vi "FlushTcpPortBase.vi"(6 "max flush time (ms)":i32=5000, 8 "error in (no error)":errorcluster, 11 "tcp in":refnum<k5>) -> (0 "error out":errorcluster, 1 "timed out":bool, 2 "data flushed":bool, 3 "tcp out":refnum<k5>)   [LabVIEW 2017]
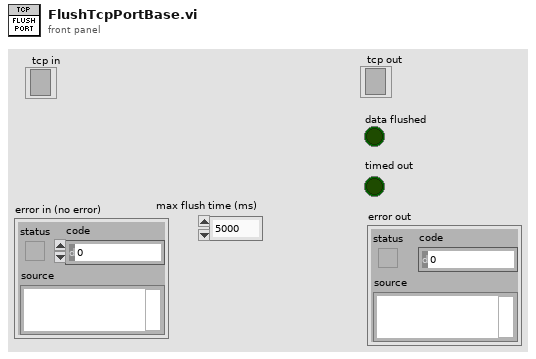
[diagram p1: front panel]
types:
  T1 = enum16{"Standard", "Buffered", "CRLF", "Immediate"}
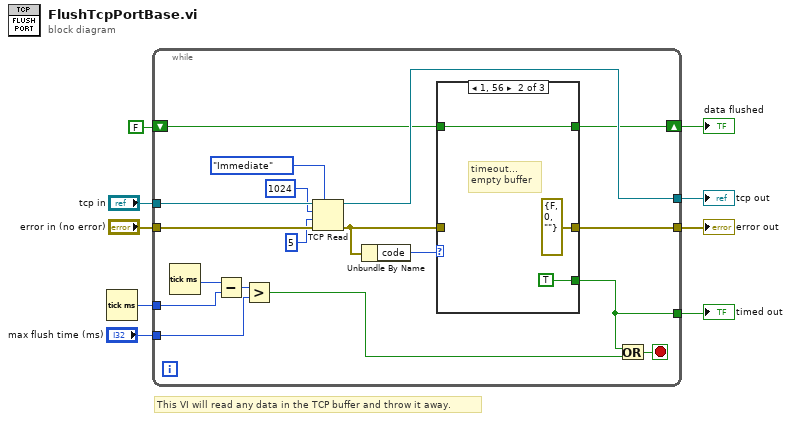
[diagram p0: block diagram]
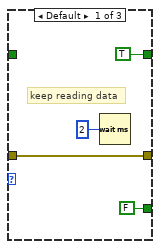
[diagram p2: hidden frame]
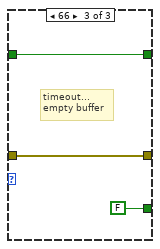
[diagram p3: hidden frame]
diagram:
  # "This VI will read any data in the TCP buffer and throw it away."
  n1 = Tick Count (ms)() -> (millisecond timer value=w3:u32)
  n2 = while {
    tunnel: "max flush time (ms)" -> [w13]
    tunnel: "tcp in" -> [w27]
    tunnel: "error in (no error)" -> [w26]
    tunnel: [w19] -> w6
    tunnel: [w18] -> w5
    tunnel: [w17] -> w4
    tunnel: w3 -> [w15]
    shift-right: [w10] -> w1
    shift-left: FALSE -> [w11]
    stop <- w20 stop-if-true
    n3 = Tick Count (ms)() -> (millisecond timer value=w16:u32)
    n4 = Subtract(x=w16, y=w15) -> (x-y=w14:u32)
    n5 = Greater?(x=w14, y=w13) -> (0:w12:bool)
    n6 = TCP Read(connection ID=w27, bytes to read=1024, error in (no error)=w26, 7:T1."Immediate" ("mode (standard)"), 9:5 ("timeout ms (25000)")) -> (connection ID out=w17:refnum<k5>, error out=w21:errorcluster)  [unwired: 1 out]
    n7 = Unbundle By Name(w21) -> ("code"=w22:i32)
    n8 = case shown="1, 56" w22 {
      tunnel: [FALSE TRUE FALSE] -> w19
      tunnel: w21 -> [w31 _ w35]
      tunnel: [w31 errorcluster {"status"=FALSE, "code"=0, "source"=""} ("error out") w35] -> w18
      tunnel: w11 -> [_ w32 w36]
      tunnel: [TRUE w32 w36] -> w10
      frame Default {
        # "keep reading data"
        n9 = Wait (ms)(milliseconds to wait=u32 2) -> ()  [unwired: 1 out]
      }
      frame 1, 56 {
        # "timeout...\nempty buffer"
      }
      frame 66 {
        # "timeout...\nempty buffer"
      }
    }
    n10 = Or(x=w19, y=w12) -> (x .or. y?=w20:bool)
  }
  "error out" <- w5
  "tcp out" <- w4
  "timed out" <- w6
  "data flushed" <- w1
